vi "Convert Heater State Enum to Shutdown Furnace.vi"(10 "Heater State":T1) -> (2 "Shutdown Furnace?":bool)   [LabVIEW 2015, in "Thermal Chamber Controller_DQMH.lvlib"]
doc: "This VI converts the Heater State enumerator to a boolean that indicates if the Furnace should be shutdown.\n____\nDelacor QMH Thermal Chamber Examples 4.0.0.21\nCopyright (c) 2018, Delacor"
uses:
  Thermal Chamber Controller_DQMH.lvlib
  Heater State--enum.ctl
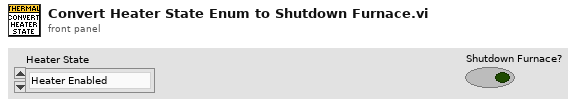
[diagram p1: front panel]
types:
  T1 = typedef "Thermal Chamber Controller_DQMH.lvlib/Heater State--enum.ctl" = enum16{"Heater Enabled", "Heater Disabled"}
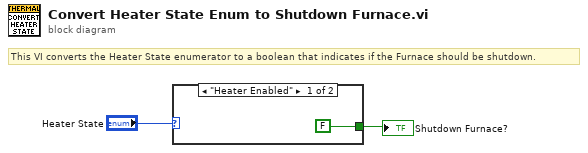
[diagram p0: block diagram]
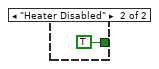
[diagram p2: hidden frame]
diagram:
  # "This VI converts the Heater State enumerator to a boolean that indicates if the Furnace should be shutdown."
  n1 = case shown="\"Heater Enabled\"" "Heater State" {
    tunnel: [FALSE ("Furnace Shutdown") TRUE ("Furnace Shutdown")] -> w2
    frame "Heater Enabled" {
    }
    frame "Heater Disabled" {
    }
  }
  "Shutdown Furnace?" <- w2
